vi "Local Configuration.Transfer Size.Set.vi"(8 "error in (no error)":errorcluster, 10 "Transfer Size":u32, 11 "GE 5565PIORC":refnum<class "GE 5565PIORC.lvclass">) -> (0 "error out":errorcluster, 3 "GE 5565PIORC out":refnum<class "GE 5565PIORC.lvclass">)   [LabVIEW 2016, in "GE 5565PIORC.lvclass"]
uses:
  GE 5565PIORC.lvclass
  Controls/Registers.Local Configuration.ctl
  GE 5565PIORC.lvclass/GE 5565PIORC.ctl
  <vilib>/Instr/_visa.llb/VISA Register Access Address Space.ctl
  Binary Operations/Get Bits U32.vi
  Binary Operations/Set Bits U32.vi
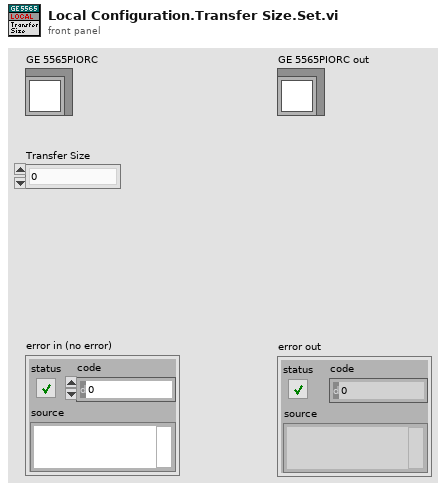
[diagram p1: front panel]
types:
  T1 = typedef "GE 5565PIORC.lvclass/Registers.Local Configuration.ctl" = enum16{"DMA Arbitration", "Interrupt Control and Status", "DMA Mode", "DMA PCI Address", "DMA Local Address", "DMA Transfer Size", "DMA Descriptor Pointer", "DMA Command/Status", "DMA PCI DAC Upper Address", "PCI PIO Address Range", "PCI PIO Base Address (Remap)"}
  T2 = typedef "VISA Register Access Address Space.ctl" = u16
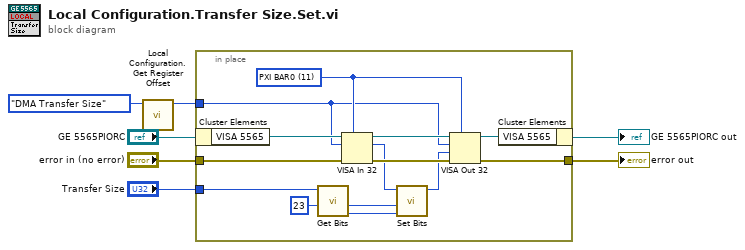
[diagram p0: block diagram]
diagram:
  n1 = call "Local Configuration.Get Register Offset.vi"("Local Configration Register"=Registers.Local_Configuration."DMA Transfer Size" ("Local Configration Register Offset")) -> ("Offset"=w1:u32)  [unwired: 10 in]
  n2 = in-place {
    in-place-border: "error in (no error)" -> [w20]
    in-place-border: [w16] -> w5
    in-place-border: "Transfer Size" -> [w9]
    in-place-border: w1 -> [w8]
    w15 = T2 11 items=["VXI/VME A16"=1, "VXI/VME A24"=2, "VXI/VME A32"=3, "VXI/VME A64"=4, "PXI Memory Allocations"=9, "PXI Configuration"=10, "PXI BAR0"=11, "PXI BAR1"=12, "PXI BAR2"=13, "PXI BAR3"=14, "PXI BAR4"=15, "PXI BAR5"=16] ("Address Space")
    n3 = in-place-cluster #1("GE 5565PIORC") -> ("VISA 5565"=w21:refnum<visa-resource-name>)
    n4 = call-poly "Get Bits.vi"("Length (1)"=u8 23, "Register in"=w9) -> ("Value"=w12:u32, "Length out"=w13:u8)  [unwired: 6 in, 2 out]
    n5 = VISA In 32(7:w15, 8:w20, 10:w8, 11:w21) -> (0:w18:errorcluster, 2:w11:u32, 3:w19:refnum<visa-resource-name>)
    n6 = call-poly "Set Bits.vi"("Value (0)"=w12, "Length (1)"=w13, "Register in"=w11) -> ("Register out"=w10:u32)  [unwired: 6 in, 2 out]
    n7 = VISA Out 32(7:w15, 8:w18, 9:w10, 10:w8, 11:w19) -> (0:w16:errorcluster, 3:w17:refnum<visa-resource-name>)
    n8 = in-place-cluster #1("VISA 5565"=w17) -> (→"GE 5565PIORC out":refnum<class "GE 5565PIORC.lvclass">)
  }
  "error out" <- w5
